vi "sendTwitterCommandResponse.vi"(8 "error in":errorcluster, 10 "TeminateOrContinue":bool, 11 "TwitterOrPanel":bool) -> (0 "error out":errorcluster, 3 "tweet sent":string)   [LabVIEW 2019]
uses:
  <vilib>/LVH/i3 Twitter/Controls/Twitter Handle.ctl
  <vilib>/LVH/i3 OAuth/Controls/OAuth Handle.ctl
  <vilib>/LVH/i3 OAuth/Controls/Signature Method.ctl
  <vilib>/LVH/i3 OAuth/Controls/Credentials.ctl
  <vilib>/LVH/i3 Twitter/SubVIs/Twitter Open - Embedded.vi
  <vilib>/LVH/i3 Twitter/Tweets/Post Tweet.vi
  <vilib>/LVH/i3 Twitter/i3-twitter.lvlib
  <vilib>/LVH/i3 OAuth/i3-oauth.lvlib
panel:
  out "Twitter Handle Out":T1={"OAuth Credentials"={"Signature Method"=enum."HMAC-SHA1", "Version"="1.0", "Client"={"Token"="", "Secret"=""}, "Access"={"Token"="", "Secret"=""}}, "since ID"="", "max ID"="", "Screen Name"=""}
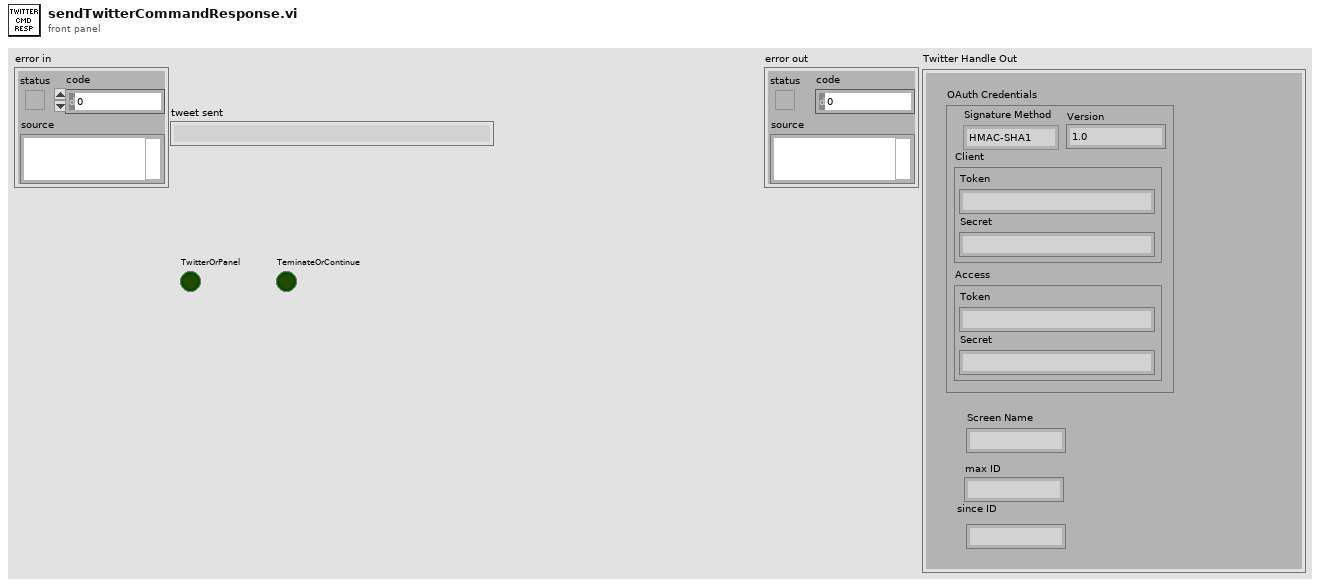
[diagram p1: front panel]
types:
  T1 = typedef "i3-twitter.lvlib/Twitter Handle.ctl" = cluster{"OAuth Credentials":T2, "since ID":string, "max ID":string, "Screen Name":string}
  T2 = typedef "i3-oauth.lvlib/OAuth Handle.ctl" = cluster{"Signature Method":T3, "Version":string, "Client":T4, "Access":T4}
  T3 = typedef "i3-oauth.lvlib/Signature Method.ctl" = enum16{"HMAC-MD5", "HMAC-SHA1", "HMAC-SHA224", "HMAC-SHA256", "HMAC-SHA384", "HMAC-SHA512"}
  T4 = typedef "i3-oauth.lvlib/Credentials.ctl" = cluster{"Token":string, "Secret":string}
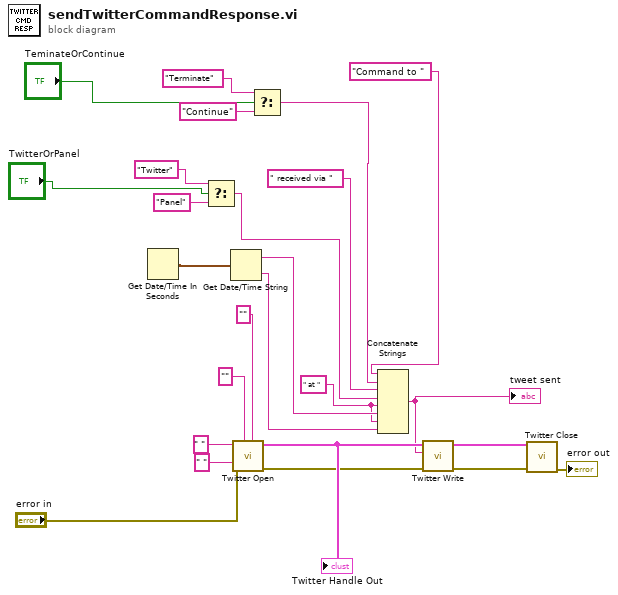
[diagram p0: block diagram]
diagram:
  w10 = " at " ("string")
  n1 = Get Date/Time In Seconds() -> (seconds since 1Jan1904=w13:timestamp)
  n2 = Select(t="Twitter" ("Tweet"), s="TwitterOrPanel", f="Panel") -> (s? t:f=w1:string)
  n3 = Get Date/Time String(seconds (now)=w13) -> (date string=w12:string, time string=w11:string)  [unwired: 2 in]
  n4 = call-poly <vilib>:"Twitter Open.vi"("Access Secret"="", "Access Token"="", "error in"="error in", "Consumer Secret"=" ", "Consumer Key"=" ") -> ("error out"=w20:errorcluster, "Twitter Handle Out"=w21:T1)  [unwired: 5 in]
  "Twitter Handle Out" <- w21
  n5 = Select(t="Terminate" ("Tweet"), s="TeminateOrContinue", f="Continue") -> (s? t:f=w5:string)
  n6 = Concatenate Strings("Command to " ("Tweet"), w5, " received via " ("Tweet"), w1, w10, w12, w10, w11) -> (w15:string)
  "tweet sent" <- w15
  n7 = call-poly <vilib>:"Twitter Write.vi"("error in (no error)"=w20, "Tweet"=w15, "Twitter Handle In"=w21) -> ("error out"=w18:errorcluster, "Twitter Handle Out"=w19:T1)  [unwired: 7 in]
  n8 = call <vilib>:"Twitter Close.vi"("error in"=w18, "Twitter Handle In"=w19) -> ("error out"=→"error out":errorcluster)  [unwired: 9 in]
